vi "Item Selection Demo.vi"() -> ()   [LabVIEW 2020, in "UI_ItemSelect_OpenSource.lvlib"]
doc: "This is a Demo VI used to demonstrate how the listbox and tree selection VIs work. Run the VI and then select items by clicking the symbols of the controls. Use Shift to select multiple items, and right click the control to use other options.\n-------------\nBrian Hoover (hooovahh)"
uses:
  UI_ItemSelect_OpenSource.lvlib
  Methods/item select new.vi
  Methods/item select select all.vi
  Methods/item select write disabled.vi
  Methods/item select read.vi
  <userlib>/_OpenG.lib/array/array.llb/Conditional Auto-Indexing Tunnel (String)__ogtk.vi
  Methods/Selection Handle Mouse Down.vi
  Methods/item select select none.vi
  Methods/item select select invert.vi
  Methods/item select destroy.vi
panel:
  out "Tree Selection":string[](array[string])
  in  "Tree":string(tree)
  out "MCLB Selection":string[](array[string])
  out "SCLB Selection":string[](array[string])
  in  "Multicolumn Listbox":i32(listbox)=-1
  in  "Listbox":i32(listbox)=-1
  # "1) Run This VI\n2) Click the checkboxes to select and unselect items.\n3) Shift can be held to change the selection of multiple items\n4) Right click the control to change the selection.\n5) Disabled items cannot be changed."
  # "Tree controls are supported with selection and deselection of parents affecting the children.  Deselecting and selecting children also will change the icon of the parent."
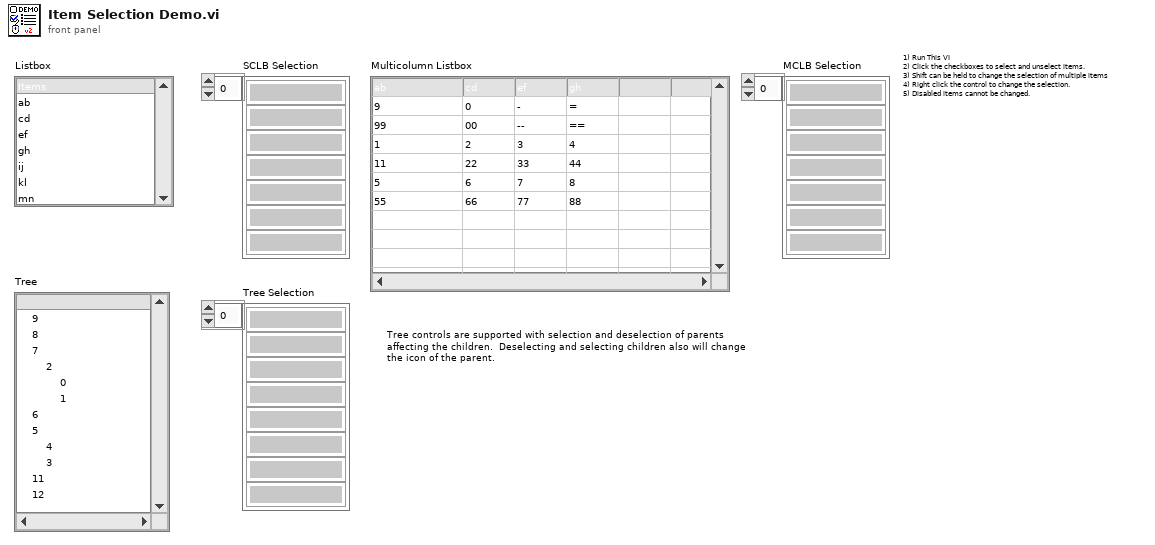
[diagram p1: front panel]
types:
  T1 = typedef "LVPoint32TypeDef.ctl" = cluster{"Horizontal":i32, "Vertical":i32}
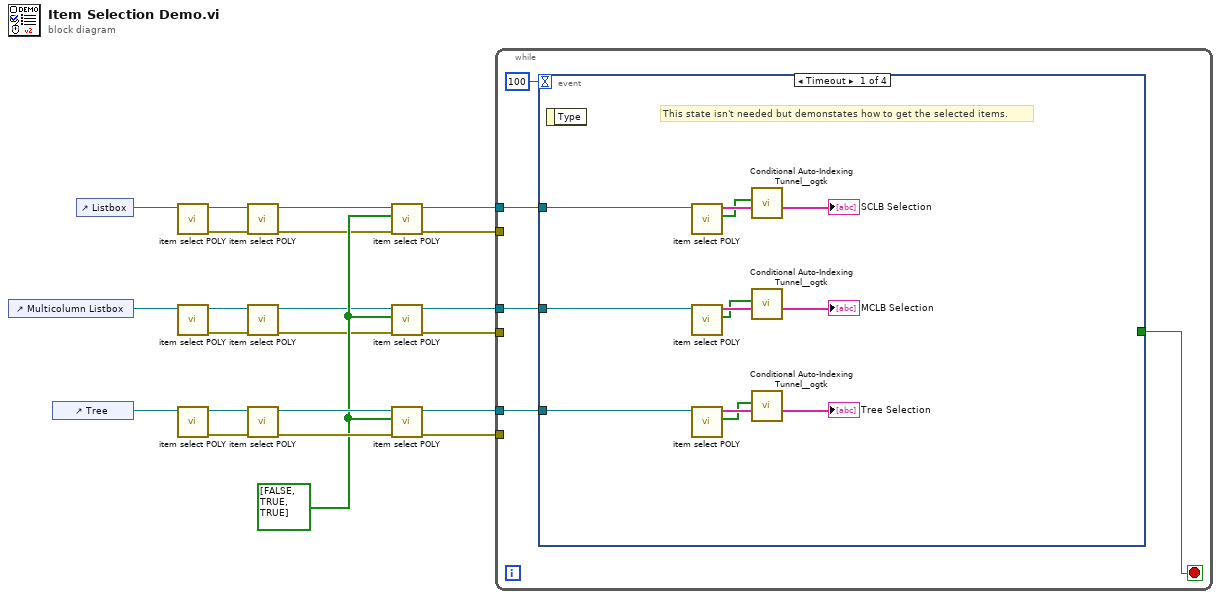
[diagram p0: block diagram]
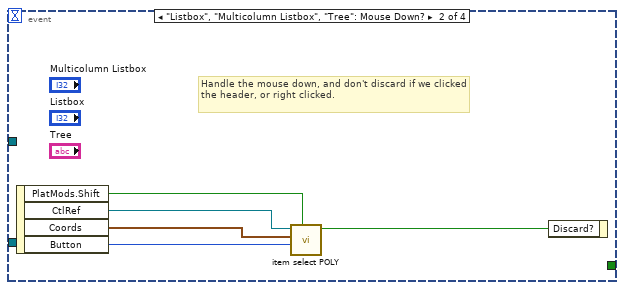
[diagram p2: hidden frame]
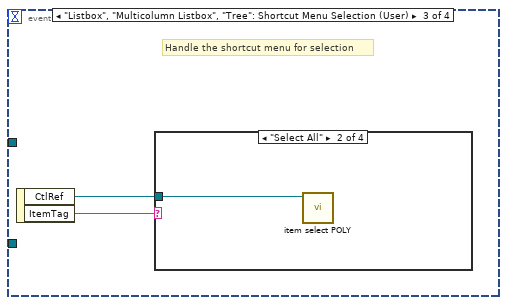
[diagram p3: hidden frame]
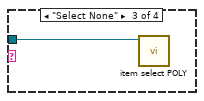
[diagram p5: hidden frame]
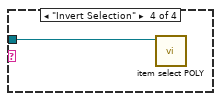
[diagram p6: hidden frame]
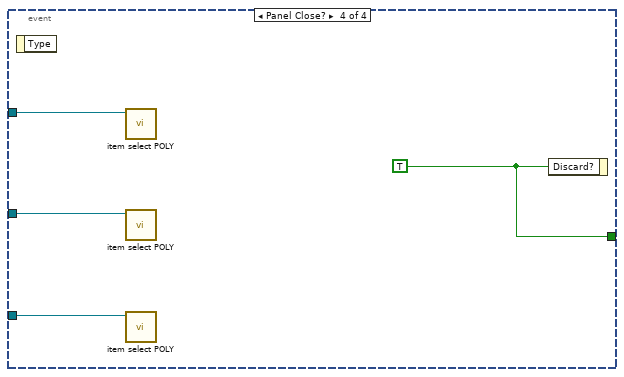
[diagram p7: hidden frame]
diagram:
  w15 = bool[] [FALSE, TRUE, TRUE] ("Disabled?")
  n1 = control-ref of="Multicolumn Listbox"() -> (w8:refnum<vi>)
  n2 = control-ref of="Tree"() -> (w1:refnum<vi>)
  n3 = control-ref of="Listbox"() -> (w9:refnum<vi>)
  n4 = call-poly "item select POLY.vi"("Listbox or Tree"=w9) -> ("error out"=w11:errorcluster, "Ref"=w7:refnum<vi>)  [unwired: 9 in]
  n5 = call-poly "item select POLY.vi"("Listbox or Tree"=w8) -> ("error out"=w10:errorcluster, "Ref"=w6:refnum<vi>)  [unwired: 9 in]
  n6 = call-poly "item select POLY.vi"("Listbox or Tree"=w1) -> ("error out"=w22:errorcluster, "Ref"=w21:refnum<vi>)  [unwired: 9 in]
  n7 = call-poly "item select POLY.vi"("error in (no error)"=w11, "Listbox or Tree"=w7) -> ("error out"=w4:errorcluster, "Ref"=w5:refnum<vi>)  [unwired: 8 in]
  n8 = call-poly "item select POLY.vi"("error in (no error)"=w10, "Listbox or Tree"=w6) -> ("error out"=w3:errorcluster, "Ref"=w2:refnum<vi>)  [unwired: 8 in]
  n9 = call-poly "item select POLY.vi"("error in (no error)"=w22, "Listbox or Tree"=w21) -> ("error out"=w20:errorcluster, "Ref"=w16:refnum<vi>)  [unwired: 8 in]
  n10 = call-poly "item select POLY.vi"("error in (no error)"=w4, "Disabled?"=w15, "Listbox or Tree"=w5) -> ("error out"=w14:errorcluster, "Ref"=w19:refnum<vi>)  [unwired: 7 in]
  n11 = call-poly "item select POLY.vi"("error in (no error)"=w3, "Disabled?"=w15, "Listbox or Tree"=w2) -> ("error out"=w13:errorcluster, "Ref"=w18:refnum<vi>)  [unwired: 7 in]
  n12 = call-poly "item select POLY.vi"("error in (no error)"=w20, "Disabled?"=w15, "Listbox or Tree"=w16) -> ("error out"=w12:errorcluster, "Ref"=w17:refnum<vi>)  [unwired: 7 in]
  n13 = while {
    tunnel: w19 -> [w25]
    tunnel: w18 -> [w24]
    tunnel: w17 -> [w23]
    tunnel: w14 -> [_]
    tunnel: w13 -> [_]
    tunnel: w12 -> [_]
    stop <- w27 stop-if-true
    n14 = event shown="[0] Timeout" {
      selector: _ -> [_ _ _ _]
      dyn-events: _ -> [_ _ _ _]
      timeout: 100 -> [_ _ _ _]
      tunnel: [_ _ _ w53] -> w27
      tunnel: w25 -> [w39 _ _ w50]
      tunnel: w24 -> [w38 _ _ w51]
      tunnel: w23 -> [w37 _ _ w52]
      event Timeout {
        # "This state isn't needed but demonstates how to get the selected items."
        n15 = event-data() -> ()  [unwired: 1 in, 1 out]
        n16 = call-poly "item select POLY.vi"("Listbox or Tree"=w39) -> ("tags.selected?"=w32:bool[], "tags.name"=w33:string[])  [unwired: 6 in, 3 out]
        n17 = call-poly "item select POLY.vi"("Listbox or Tree"=w38) -> ("tags.selected?"=w29:bool[], "tags.name"=w30:string[])  [unwired: 6 in, 3 out]
        n18 = call-poly "item select POLY.vi"("Listbox or Tree"=w37) -> ("tags.selected?"=w35:bool[], "tags.name"=w36:string[])  [unwired: 6 in, 3 out]
        n19 = call-poly <userlib>:"Conditional Auto-Indexing Tunnel__ogtk.vi"("Array in"=w33, "Elements to keep"=w32) -> ("Filtered Array out"=→"SCLB Selection":string[])  [unwired: 5 in]
        n20 = call-poly <userlib>:"Conditional Auto-Indexing Tunnel__ogtk.vi"("Array in"=w30, "Elements to keep"=w29) -> ("Filtered Array out"=→"MCLB Selection":string[])  [unwired: 5 in]
        n21 = call-poly <userlib>:"Conditional Auto-Indexing Tunnel__ogtk.vi"("Array in"=w36, "Elements to keep"=w35) -> ("Filtered Array out"=→"Tree Selection":string[])  [unwired: 5 in]
      }
      event "Listbox", "Multicolumn Listbox", "Tree": Mouse Down? {
        # "Handle the mouse down, and don't discard if we clicked the header, or right clicked."
        n22 = event-data() -> ("PlatMods.Shift"=w41:bool, "CtlRef"=w44:refnum<vi>, "Coords"=w43:T1, "Button"=w42:u16)  [unwired: 1 in]
        n23 = call-poly "item select POLY.vi"("Shift?"=w41, "Mouse Button"=w42, "Mouse Coords"=w43, "Listbox or Tree"=w44) -> ("Discard?"=w40:bool)  [unwired: 6 in, 1 out]
        n24 = event-data("Discard?"=w40) -> ()  [unwired: 1 in, 1 out]
      }
      event "Listbox", "Multicolumn Listbox", "Tree": Shortcut Menu Selection (User) {
        # "Handle the shortcut menu for selection"
        n25 = event-data() -> ("CtlRef"=w46:refnum<vi>, "ItemTag"=w45:string)  [unwired: 1 in]
        n26 = case shown="\"Select All\"" w45 {
          tunnel: w46 -> [_ w47 w48 w49]
          frame Default {
          }
          frame "Select All" {
            n27 = call-poly "item select POLY.vi"("Listbox or Tree"=w47) -> ()  [unwired: 9 in, 2 out]
          }
          frame "Select None" {
            n28 = call-poly "item select POLY.vi"("Listbox or Tree"=w48) -> ()  [unwired: 9 in, 2 out]
          }
          frame "Invert Selection" {
            n29 = call-poly "item select POLY.vi"("Listbox or Tree"=w49) -> ()  [unwired: 9 in, 2 out]
          }
        }
      }
      event Panel Close? {
        w53 = TRUE ("Discard?")
        n30 = event-data() -> ()  [unwired: 1 in, 1 out]
        n31 = call-poly "item select POLY.vi"("Listbox or Tree"=w50) -> ()  [unwired: 10 in, 1 out]
        n32 = call-poly "item select POLY.vi"("Listbox or Tree"=w51) -> ()  [unwired: 10 in, 1 out]
        n33 = call-poly "item select POLY.vi"("Listbox or Tree"=w52) -> ()  [unwired: 10 in, 1 out]
        n34 = event-data("Discard?"=w53) -> ()  [unwired: 1 in, 1 out]
      }
    }
  }
